vi "Create DataColumn.vi"(8 "错误输入（无错误）":errorcluster, 10 "DataType":variant, 11 "columnName":string) -> (0 "错误输出":errorcluster, 3 "DataColumn":refnum<k24>)   [LabVIEW 2012, in "DataGridView.lvlib"]
uses:
  DataGridView.lvlib
  System.Data
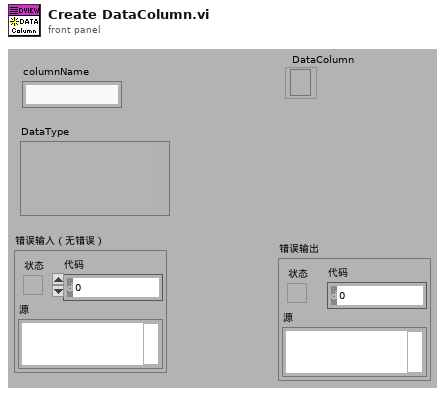
[diagram p1: front panel]
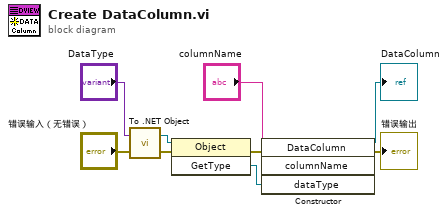
[diagram p0: block diagram]
diagram:
  n1 = call <vilib>:"To .NET Object.vi"("error in (no error)"="错误输入（无错误）", "anything"="DataType") -> ("error out"=w8:errorcluster, ".NET object"=w7:refnum<k24>)
  n2 = invoke class="Object" method="GetType"(reference=w7, error in=w8) -> (error out=w2:errorcluster, "GetType"=w6:refnum<k24>)  [unwired: 1 in, 1 out]
  n3 = constructor class="DataColumn"(error in=w2, "columnName"="columnName", "dataType"=w6) -> (reference out=→"DataColumn":refnum<k24>, error out=→"错误输出":errorcluster)  [unwired: 2 in, 3 out]
